vi "Load RSL File.vi"(8 "error in (no error)":errorcluster, 11 "RSL Path":path) -> (0 "error out":errorcluster, 2 "invalid file?":bool, 3 "RSL Data":T9 {"Test Config Data"."Test Ranking" items=["Low", "Normal", "High"]})   [LabVIEW 2019]
uses:
  <vilib>/addons/analyzer/_analyzerctrls.llb/VIAnCtl Results.ctl
  <vilib>/addons/analyzer/_analyzerctrls.llb/VIAnCtl ResultsData (index).ctl
  <vilib>/addons/analyzer/_analyzerctrls.llb/VIAnCtl ResultStatus.ctl
  <vilib>/addons/analyzer/_vianresshared.llb/VIAnRes Parsed Results Data (by VI).ctl
  <vilib>/addons/analyzer/_vianresshared.llb/VIAnRes Parsed Results Data (by Test).ctl
  <vilib>/addons/analyzer/_analyzerctrls.llb/VIAnCtl Test Config Data.ctl
  <vilib>/addons/analyzer/_analyzerctrls.llb/VIAnCtl TestRanking.ctl
  <vilib>/addons/analyzer/_analyzerctrls.llb/VIAnCtl Config Control Value.ctl
panel:
  in  "old rsl":string="This RSL file was saved with LabVIEW 2017 or previous. Object highlighting in the VI Analyzer Results Window is not supported with older RSL files in LabVIEW 2018 and later."
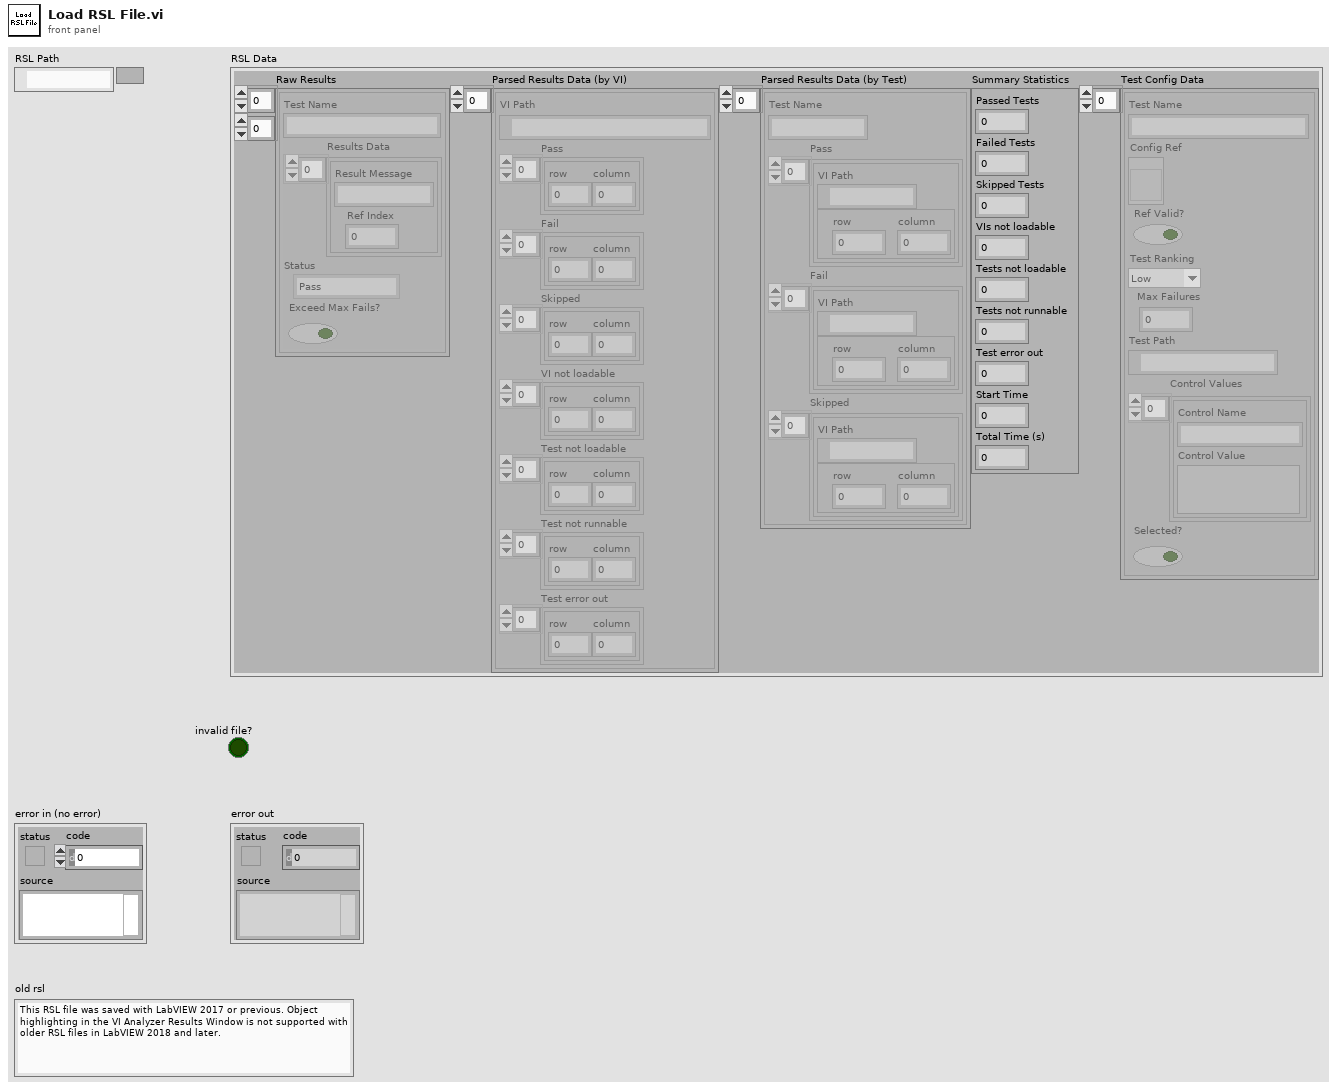
[diagram p1: front panel]
types:
  T1 = typedef "VIAnCtl Results.ctl" = cluster{"Test Name":string, "Results Data":T2[], "Status":T3, "Exceed Max Fails?":bool}
  T2 = typedef "VIAnCtl ResultsData (index).ctl" = cluster{"Result Message":string, "Ref Index":i32}
  T3 = typedef "VIAnCtl ResultStatus.ctl" = enum16{"Pass", "Fail", "Skipped", "VI not loadable", "Test not loadable", "Test not runnable", "Test error out"}
  T4 = typedef "VIAnRes Parsed Results Data (by VI).ctl" = cluster{"VI Path":path, "Pass":cluster{"row":i32, "column":i32}[], "Fail":cluster{"row":i32, "column":i32}[], "Skipped":cluster{"row":i32, "column":i32}[], "VI not loadable":cluster{"row":i32, "column":i32}[], "Test not loadable":cluster{"row":i32, "column":i32}[], "Test not runnable":cluster{"row":i32, "column":i32}[], "Test error out":cluster{"row":i32, "column":i32}[]}
  T5 = typedef "VIAnRes Parsed Results Data (by Test).ctl" = cluster{"Test Name":string, "Pass":cluster{"VI Path":path, "index":cluster{"row":i32, "column":i32}}[], "Fail":cluster{"VI Path":path, "index":cluster{"row":i32, "column":i32}}[], "Skipped":cluster{"VI Path":path, "index":cluster{"row":i32, "column":i32}}[]}
  T6 = typedef "VIAnCtl Test Config Data.ctl" = cluster{"Test Name":string, "Config Ref":refnum<vi>, "Ref Valid?":bool, "Test Ranking":T7, "Max Failures":u32, "Test Path":path, "Control Values":T8[], "Selected?":bool}
  T7 = typedef "VIAnCtl TestRanking.ctl" = u16
  T8 = typedef "VIAnCtl Config Control Value.ctl" = cluster{"Control Name":string, "Control Value":variant}
  T9 = cluster{"Raw Results":T1[][], "Parsed Results Data (by VI)":T4[], "Parsed Results Data (by Test)":T5[], "Summary Statistics":cluster{"Passed Tests":i32, "Failed Tests":i32, "Skipped Tests":i32, "VIs not loadable":i32, "Tests not loadable":i32, "Tests not runnable":i32, "Test error out":i32, "Start Time":u32, "Total Time (s)":dbl}, "Test Config Data":T6[]}
  T10 = cluster{"Passed Tests":i32, "Failed Tests":i32, "Skipped Tests":i32, "VIs not loadable":i32, "Tests not loadable":i32, "Tests not runnable":i32, "Test error out":i32, "Start Time":u32, "Total Time (s)":dbl}
  T11 = cluster{"Pass":i32, "Fail":i32, "Skipped":i32, "VI not loadable":i32, "Test not loadable":i32, "Test not runnable":i32, "Test error out":i32}
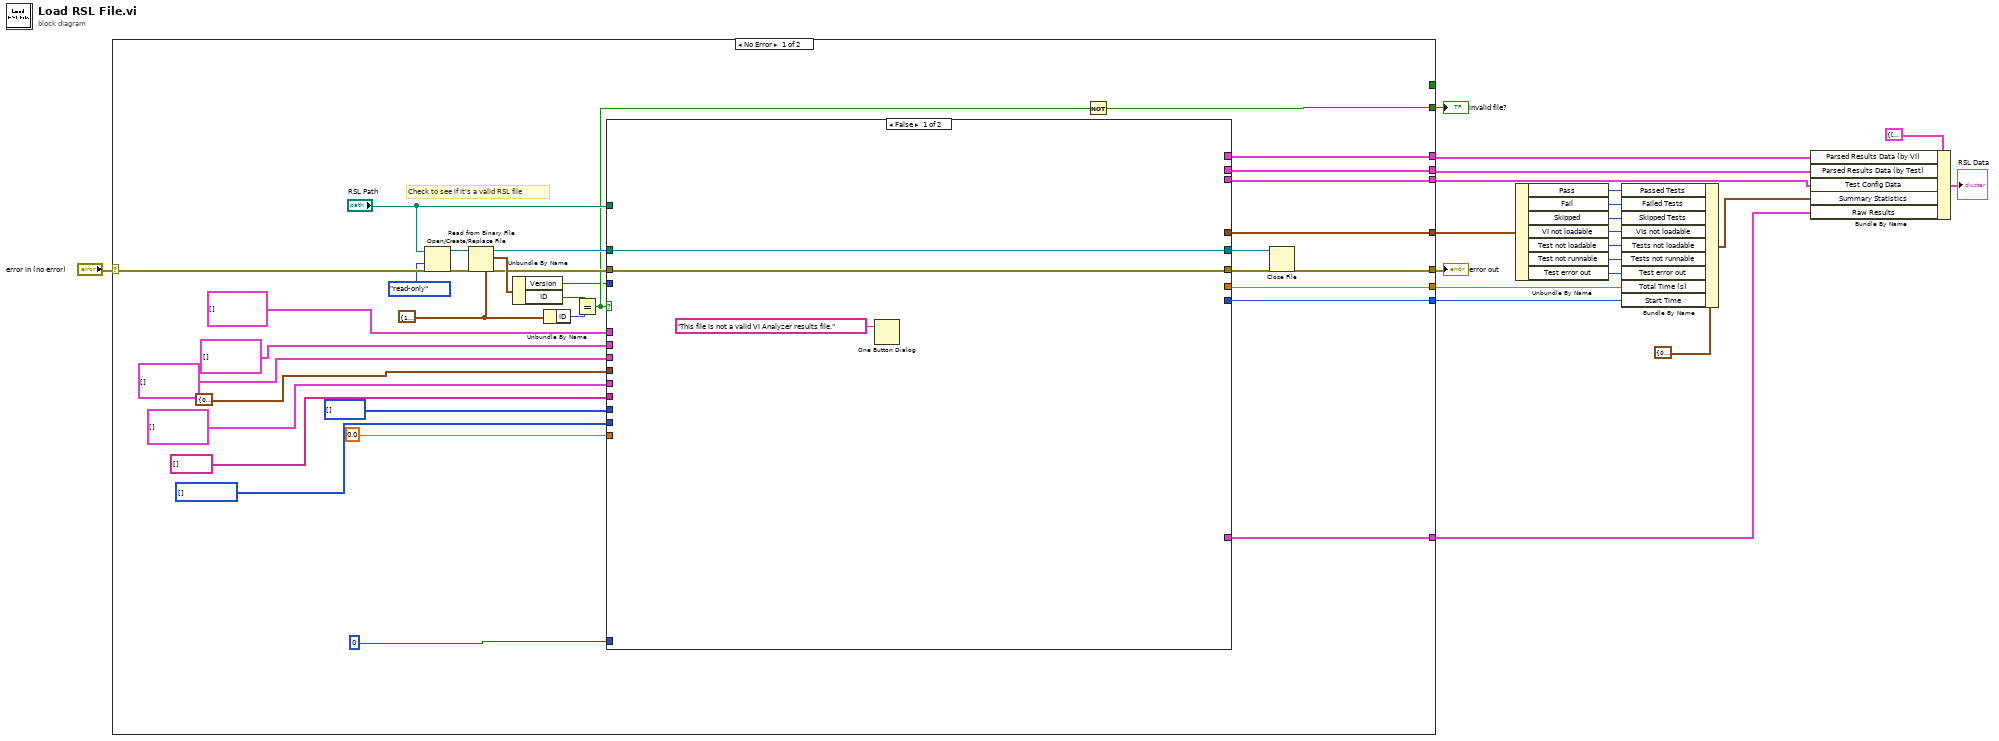
[diagram p0: block diagram]
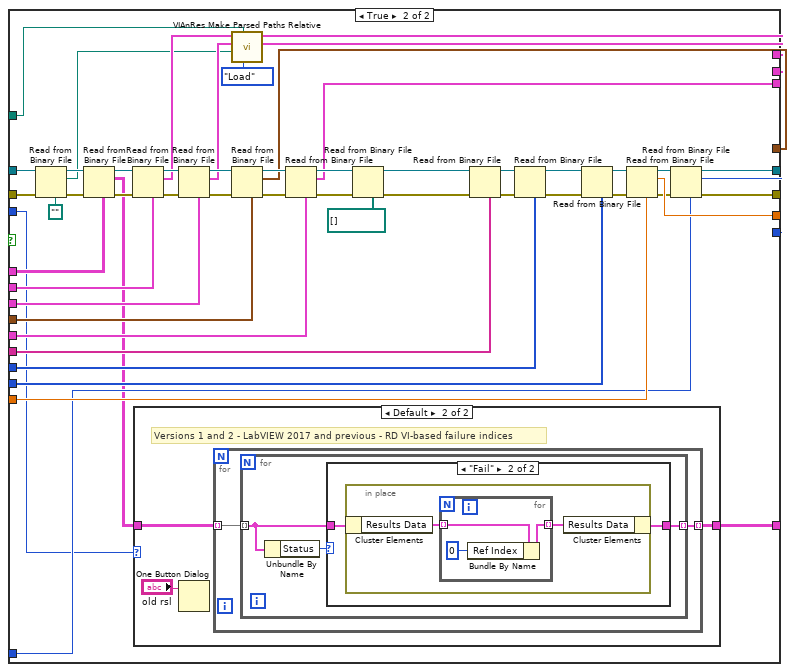
[diagram p2: hidden frame]
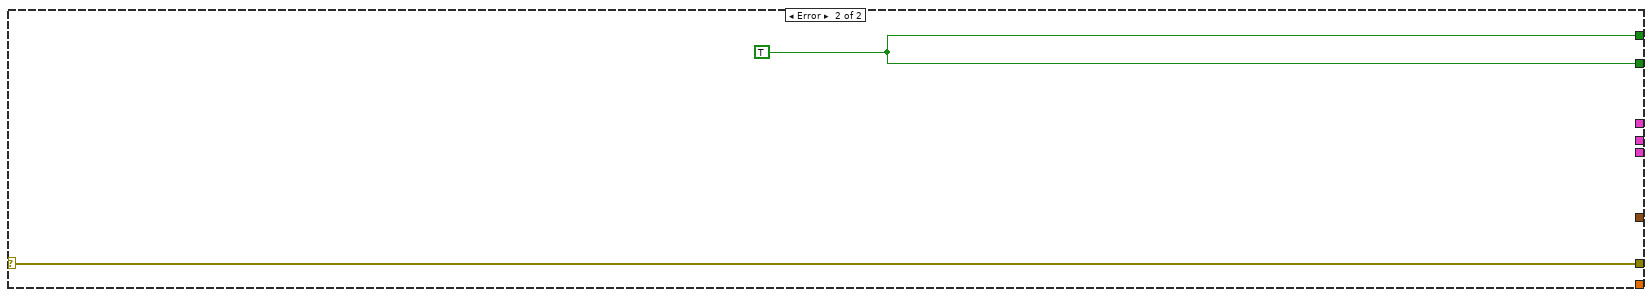
[diagram p5: hidden frame]
diagram:
  n1 = case shown="No Error" "error in (no error)" {
    selector: "error in (no error)" -> [w48 w129]
    tunnel: [w55 w129] -> w20
    tunnel: [_ w128] -> _
    tunnel: [w54 w128] -> w19
    tunnel: [w53 _] -> w17
    tunnel: [w52 _] -> w16
    tunnel: [w51 _] -> w14
    tunnel: [w50 _] -> w5
    tunnel: [w49 _] -> w6
    tunnel: [w47 _] -> w4
    tunnel: [w46 _] -> w2
    frame No Error {
      w22 = cluster{"ID":i32, "Version":i32} {"ID"=1934326086, "Version"=3} ("File Info")
      w39 = T7[] [] items=["Low", "Normal", "High"] ("dum Rankings")
      # "Check to see if it's a valid RSL file"
      n2 = Open/Create/Replace File(file path (use dialog)="RSL Path", error in=w48, access (0:read/write)=enum16{"read/write", "read-only", "write-only"}."read-only") -> (refnum out=w24:refnum<file>, error out=w25:errorcluster)  [unwired: 4 out]
      n3 = Read from Binary File ("Read File")(5:w22, 8:w25, 11:w24) -> (0:w31:errorcluster, 2:w34:cluster{"ID":i32, "Version":i32}, 3:w30:refnum<file>)  [unwired: 4 out]
      n4 = Unbundle By Name(w34) -> ("Version"=w23:i32, "ID"=w33:i32)
      n5 = Unbundle By Name(w22) -> ("ID"=w32:i32)
      n6 = Equal?(x=w33, y=w32) -> (x = y?=w29:bool)
      n7 = case shown="False" w29 {
        tunnel: w31 -> [w57 w69]
        tunnel: w30 -> [w58 w68]
        tunnel: [w57 w89] -> w27
        tunnel: T4[] [] ("dum Parsed Results Data (by VI)") -> [_ w110]
        tunnel: T5[] [] ("dum Parsed Results Data (by Test)") -> [_ w109]
        tunnel: T11 {"Pass"=0, "Fail"=0, "Skipped"=0, "VI not loadable"=0, "Test not loadable"=0, "Test not runnable"=0, "Test error out"=0} ("dum Numbers") -> [_ w106]
        tunnel: T6[] [] ("dum Test Config Data") -> [_ w103]
        tunnel: u32[] [] ("dum Max Failures") -> [_ w102]
        tunnel: [w58 w88] -> w28
        tunnel: string[] [] ("dum Tags") -> [_ w99]
        tunnel: w39 -> [_ w94]
        tunnel: [_ w72] -> w53
        tunnel: [_ w71] -> w52
        tunnel: [_ w75] -> w51
        tunnel: 0.0 ("dum Tot Time") -> [_ w91]
        tunnel: [_ w90] -> w50
        tunnel: [_ w85] -> w49
        tunnel: u32 0 ("dum Timestamp") -> [_ w84]
        tunnel: "RSL Path" -> [_ w63]
        tunnel: T1[][] [] ("dum Raw Data") -> [_ w81]
        tunnel: w23 -> [_ w62]
        tunnel: [_ w60] -> w47
        tunnel: [_ w59] -> w46
        frame False {
          n8 = One Button Dialog(message="This file is not a valid VI Analyzer results file.") -> ()  [unwired: 2 out]
        }
        frame True {
          n9 = Read from Binary File ("Read File")(5:path "", 8:w69, 11:w68) -> (0:w66:errorcluster, 2:w64:path, 3:w67:refnum<file>)  [unwired: 4 out]
          n10 = Read from Binary File ("Read File")(5:w81, 8:w66, 11:w67) -> (0:w82:errorcluster, 2:w61:T1[][], 3:w83:refnum<file>)  [unwired: 4 out]
          n11 = Read from Binary File ("Read File")(5:w110, 8:w82, 11:w83) -> (0:w97:errorcluster, 2:w74:T4[], 3:w98:refnum<file>)  [unwired: 4 out]
          n12 = case shown="Default" w62 {
            tunnel: [w111 w113] -> w60
            tunnel: w61 -> [w111 w114]
            frame 3 {
              # "Version 3 - LabVIEW 2018 and later - UIDs for object failures"
            }
            frame Default {
              # "Versions 1 and 2 - LabVIEW 2017 and previous - RD VI-based failure indices"
              n13 = One Button Dialog(message="old rsl") -> ()  [unwired: 1 in, 1 out]
              n14 = for {
                tunnel: w114 -> [w116] mode=indexing
                tunnel: [w115] -> w113 mode=indexing
                n15 = for {
                  tunnel: w116 -> [w118] mode=indexing
                  tunnel: [w117] -> w115 mode=indexing
                  n16 = Unbundle By Name(w118) -> ("Status"=w119:T3)
                  n17 = case shown="\"Fail\"" w119 {
                    tunnel: w118 -> [w120 w122]
                    tunnel: [w120 w121] -> w117
                    frame Default {
                    }
                    frame "Fail" {
                      n18 = in-place {
                        n19 = in-place-cluster #1(w122) -> ("Results Data"=w124:T2[])
                        n20 = for {
                          tunnel: w124 -> [w127] mode=indexing
                          tunnel: [w126] -> w123 mode=indexing
                          n21 = Bundle By Name(cluster=w127, "Ref Index"=0) -> (w126:T2)
                        }
                        n22 = in-place-cluster #1("Results Data"=w123) -> (w121:T1)
                      }
                    }
                  }
                }
              }
            }
          }
          n23 = Read from Binary File ("Read File")(5:w109, 8:w97, 11:w98) -> (0:w107:errorcluster, 2:w73:T5[], 3:w108:refnum<file>)  [unwired: 4 out]
          n24 = call <vilib>:"VIAnRes Make Parsed Paths Relative.vi"("Op"=enum16{"Load", "Save"}."Load", "Current RSL Path"=w63, "Stored RSL Path"=w64, "Parsed Results Data (by Test) in"=w73, "Parsed Results Data (by VI) in"=w74) -> ("Parsed Results Data (by Test) out"=w71:T5[], "Parsed Results Data (by VI) out"=w72:T4[])  [unwired: 5 out]
          n25 = Read from Binary File ("Read File")(5:w106, 8:w107, 11:w108) -> (0:w104:errorcluster, 2:w75:T11, 3:w105:refnum<file>)  [unwired: 4 out]
          n26 = Read from Binary File ("Read File")(5:w103, 8:w104, 11:w105) -> (0:w79:errorcluster, 2:w59:T6[], 3:w80:refnum<file>)  [unwired: 4 out]
          n27 = Read from Binary File ("Read File")(5:path[] [], 8:w79, 11:w80) -> (0:w77:errorcluster, 3:w78:refnum<file>)  [unwired: 5 out]
          n28 = Read from Binary File ("Read File")(5:w99, 8:w77, 11:w78) -> (0:w100:errorcluster, 3:w101:refnum<file>)  [unwired: 5 out]
          n29 = Read from Binary File ("Read File")(5:w102, 8:w100, 11:w101) -> (0:w95:errorcluster, 3:w96:refnum<file>)  [unwired: 5 out]
          n30 = Read from Binary File ("Read File")(5:w94, 8:w95, 11:w96) -> (0:w92:errorcluster, 3:w93:refnum<file>)  [unwired: 5 out]
          n31 = Read from Binary File ("Read File")(5:w91, 8:w92, 11:w93) -> (0:w86:errorcluster, 2:w90:dbl, 3:w87:refnum<file>)  [unwired: 4 out]
          n32 = Read from Binary File ("Read File")(5:w84, 8:w86, 11:w87) -> (0:w89:errorcluster, 2:w85:u32, 3:w88:refnum<file>)  [unwired: 4 out]
        }
      }
      n33 = Not(x=w29) -> (.not. x?=w54:bool)
      n34 = Close File(refnum=w28, error in=w27) -> (error out=w55:errorcluster)  [unwired: 1 out]
    }
    frame Error {
      w128 = TRUE
    }
  }
  "error out" <- w20
  "invalid file?" <- w19
  n35 = Unbundle By Name(w14) -> ("Pass"=w7:i32, "Fail"=w8:i32, "Skipped"=w9:i32, "VI not loadable"=w10:i32, "Test not loadable"=w13:i32, "Test not runnable"=w12:i32, "Test error out"=w11:i32)
  n36 = Bundle By Name(cluster=T10 {"Passed Tests"=0, "Failed Tests"=0, "Skipped Tests"=0, "VIs not loadable"=0, "Tests not loadable"=0, "Tests not runnable"=0, "Test error out"=0, "Start Time"=0, "Total Time (s)"=0.0} ("Summary Statistics"), "Passed Tests"=w7, "Failed Tests"=w8, "Skipped Tests"=w9, "VIs not loadable"=w10, "Tests not loadable"=w13, "Tests not runnable"=w12, "Test error out"=w11, "Total Time (s)"=w5, "Start Time"=w6) -> (w3:T10)
  n37 = Bundle By Name(cluster=T9 {"Raw Results"=[], "Parsed Results Data (by VI)"=[], "Parsed Results Data (by Test)"=[], "Summary Statistics"={"Passed Tests"=0, "Failed Tests"=0, "Skipped Tests"=0, "VIs not loadable"=0, "Tests not loadable"=0, "Tests not runnable"=0, "Test error out"=0, "Start Time"=0, "Total Time (s)"=0.0}, "Test Config Data"=[]} ("Analysis Results"), "Parsed Results Data (by VI)"=w17, "Parsed Results Data (by Test)"=w16, "Test Config Data"=w2, "Summary Statistics"=w3, "Raw Results"=w4) -> (→"RSL Data":T9)
